vi "_rep_cap_get_nameIDs_range.vi"(7 "RepCap value in":variant, 8 "error in":errorcluster caption="error in (no error)", 11 "RepCap Type in":T1) -> (0 "error out":errorcluster, 2 "First NameID out":string, 3 "ID range out":string)   [LabVIEW 2022 SP3, in "hmp4000_rsidr_core.lvlib"]
uses:
  hmp4000_rsidr_core.lvlib
  _type_RepCap_Type.ctl
  Trim Whitespace One-Sided.vi
  Match Regular Expression.xnode
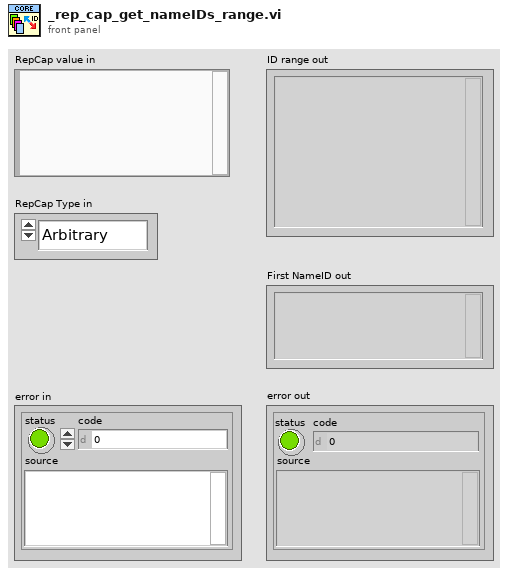
[diagram p1: front panel]
types:
  T1 = typedef "hmp4000_rsidr_core.lvlib/_type_RepCap_Type.ctl" = enum16{"Arbitrary", "SequentialNull", "Sequential"}
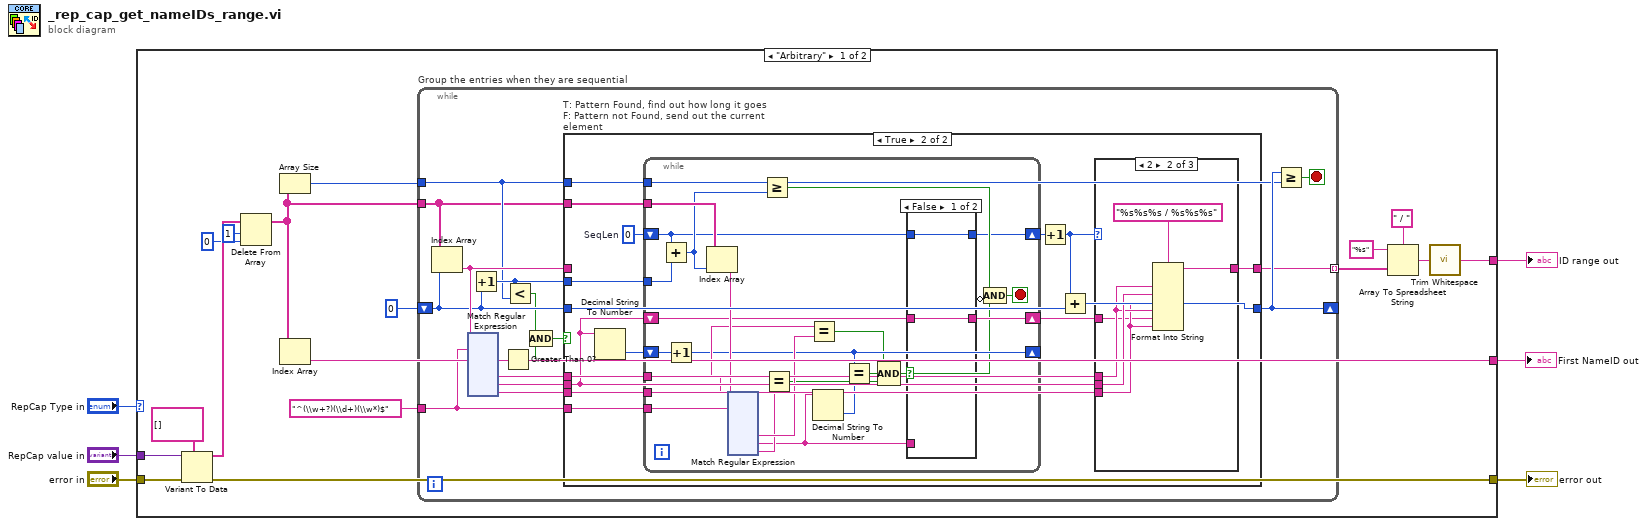
[diagram p0: block diagram]
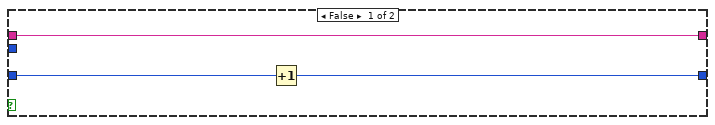
[diagram p2: hidden frame]
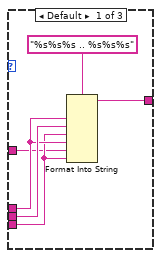
[diagram p3: hidden frame]
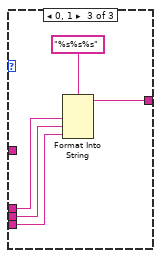
[diagram p4: hidden frame]
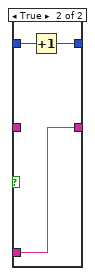
[diagram p5: hidden frame]
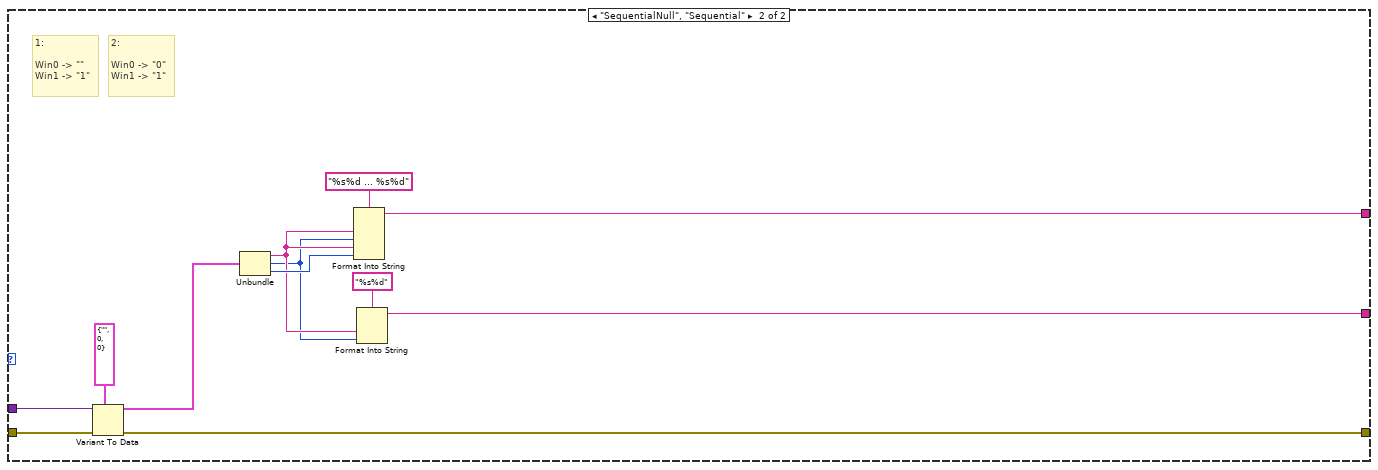
[diagram p6: hidden frame]
diagram:
  n1 = case shown="\"Arbitrary\"" "RepCap Type in" {
    tunnel: [w10 w354] -> w6
    tunnel: "RepCap value in" -> [w22 w356]
    tunnel: "error in" -> [w23 w357]
    tunnel: [w20 w350] -> w3
    tunnel: [w8 w346] -> w1
    frame "Arbitrary" {
      n2 = Variant To Data(error in=w23, type=string[] [], Variant=w22) -> (data=w19:string[], error out=w20:errorcluster)
      n3 = Delete From Array(array=w19, length=1, index=0) -> (array with subset deleted=w7:string[])  [unwired: 1 out]
      n4 = Array Size(array=w7) -> (size(s)=w16:i32)
      n5 = Index Array(array=w7) -> (element=w8:string)  [unwired: 1 in]
      n6 = while "Group the entries when they are sequential" {
        shift-right: [w38] -> _
        shift-left: 0 -> [w31]
        tunnel: w7 -> [w25]
        tunnel: "^(\\w+?)(\\d+)(\\w*)$" ("regular expression") -> [w24]
        tunnel: w16 -> [w26]
        tunnel: [w35] -> w11 mode=indexing
        stop <- w37 stop-if-true
        n7 = Index Array(array=w25, index=w31) -> (element=w36:string)
        n8 = xnode ("Match Regular Expression")("input string"=w36, "regular expression"=w24) -> ("offset past match"=w39:i32, "submatch 1"=w34:string, "submatch 2"=w33:string, "submatch 3"=w32:string)  [unwired: 4 in, 4 out]
        n9 = Increment(x=w31) -> (x+1=w27:i32)
        n10 = Greater Than 0?(x=w39) -> (x > 0?=w30:bool)
        n11 = Less?(x=w27, y=w26) -> (x < y?=w28:bool)
        n12 = Compound Arithmetic op=AND(w28, w30) -> (w29:bool)
        n13 = case "T: Pattern Found, find out how long it goes\nF: Pattern not Found, send out the current element" shown="True" w29 {
          tunnel: w31 -> [w42 w46]
          tunnel: [w41 w45] -> w38
          tunnel: w36 -> [w40 _]
          tunnel: [w40 w47] -> w35
          tunnel: w34 -> [_ w54]
          tunnel: w33 -> [_ w51]
          tunnel: w32 -> [_ w52]
          tunnel: w27 -> [_ w49]
          tunnel: w26 -> [_ w57]
          tunnel: w25 -> [_ w56]
          tunnel: w24 -> [_ w53]
          frame False {
            n14 = Increment(x=w42) -> (x+1=w41:i32)
          }
          frame True {
            w48 = 0  # SeqLen
            n15 = Decimal String To Number(string=w51) -> (number=w55:i32)  [unwired: 2 in, 1 out]
            n16 = while {
              tunnel: w54 -> [w93]
              tunnel: w52 -> [w91]
              tunnel: w57 -> [w98]
              tunnel: w56 -> [w97]
              tunnel: w53 -> [w94]
              shift-right: [w87] -> _
              shift-left: w55 -> [w89]
              shift-right: [w76] -> w50
              shift-left: w51 -> [w77]
              shift-right: [w79] -> w44
              shift-left: w48 -> [w80]
              tunnel: w49 -> [w81]
              stop <- w82 stop-if-true
              n17 = Add(x=w80, y=w81) -> (x+y=w96:i32)
              n18 = Increment(x=w89) -> (x+1=w87:i32)
              n19 = Index Array(array=w97, index=w96) -> (element=w95:string)
              n20 = xnode ("Match Regular Expression")("input string"=w95, "regular expression"=w94) -> ("submatch 1"=w92:string, "submatch 2"=w78:string, "submatch 3"=w90:string)  [unwired: 4 in, 5 out]
              n21 = Greater Or Equal?(x=w98, y=w96) -> (x >= y?=w83:bool)
              n22 = Equal?(x=w91, y=w90) -> (x = y?=w84:bool)
              n23 = Equal?(x=w93, y=w92) -> (x = y?=w86:bool)
              n24 = Decimal String To Number(string=w78) -> (number=w88:i32)  [unwired: 2 in, 1 out]
              n25 = Equal?(x=w87, y=w88) -> (x = y?=w85:bool)
              n26 = Compound Arithmetic op=AND(w86, w85, w84) -> (w75:bool)
              n27 = case shown="False" w75 {
                tunnel: w80 -> [w100 w103]
                tunnel: [w100 w102] -> w79
                tunnel: w78 -> [_ w101]
                tunnel: w77 -> [w99 _]
                tunnel: [w99 w101] -> w76
                frame False {
                }
                frame True {
                  n28 = Increment(x=w103) -> (x+1=w102:i32)
                }
              }
              n29 = Compound Arithmetic op=AND(w83, invert w75) -> (w82:bool)
            }
            n30 = Increment(x=w44) -> (x+1=w43:i32)
            n31 = Add(x=w43, y=w46) -> (x+y=w45:i32)
            n32 = case shown="2" w43 {
              tunnel: w54 -> [w60 w66 w71]
              tunnel: w52 -> [w59 w65 w70]
              tunnel: w51 -> [w62 w68 w73]
              tunnel: w50 -> [w58 w64 _]
              tunnel: [w61 w67 w72] -> w47
              frame Default {
                n33 = Format Into String(format string="%s%s%s .. %s%s%s", w60, w62, w59, w60, w58, w59) -> (resulting string=w61:string)  [unwired: 2 in, 1 out]
              }
              frame 2 {
                n34 = Format Into String(format string="%s%s%s / %s%s%s", w66, w68, w65, w66, w64, w65) -> (resulting string=w67:string)  [unwired: 2 in, 1 out]
              }
              frame 0, 1 {
                n35 = Format Into String(format string="%s%s%s", w71, w73, w70) -> (resulting string=w72:string)  [unwired: 2 in, 1 out]
              }
            }
          }
        }
        n36 = Greater Or Equal?(x=w38, y=w26) -> (x >= y?=w37:bool)
      }
      n37 = Array To Spreadsheet String(delimiter (Tab)=" / ", array=w11, 3:"%s" ("format string")) -> (spreadsheet string=w12:string)
      n38 = call "Trim Whitespace.vi"("string"=w12) -> ("trimmed string"=w10:string)  [unwired: 1 in]
    }
    frame "SequentialNull", "Sequential" {
      # "1:\n\nWin0 -> \"\"\nWin1 -> \"1\""
      # "2:\n\nWin0 -> \"0\"\nWin1 -> \"1\""
      n39 = Variant To Data(error in=w357, type=cluster{string, i32, i32} {"", 0, 0} ("output cluster"), Variant=w356) -> (data=w352:cluster{string, i32, i32}, error out=w350:errorcluster)
      n40 = Unbundle(w352) -> (w348:string, w347:i32, w355:i32)
      n41 = Format Into String(format string="%s%d ... %s%d" ("error message (\"\")"), w348, w347, w348, w355) -> (resulting string=w354:string)  [unwired: 2 in, 1 out]
      n42 = Format Into String(format string="%s%d", w348, w347) -> (resulting string=w346:string)  [unwired: 2 in, 1 out]
    }
  }
  "ID range out" <- w6
  "error out" <- w3
  "First NameID out" <- w1
